vi "Actor Core.vi"(8 "error in":errorcluster, 11 "Aumentar_contador in":refnum<class "Aumentar_contador.lvclass">) -> (0 "error out":errorcluster, 3 "Actor out":refnum<class "Actor.lvclass">)   [LabVIEW 2019, in "Aumentar_contador.lvlib" / "Aumentar_contador.lvclass"]
doc: "(<B>Filename</B>: Actor Framework.lvlib:Actor.lvclass:Actor Core.vi)\n\nReceives messages to the actor, reacts to them, and initiates any error handling that may shut the actor down.\n\nDescendant classes may override this VI to append parallel tasks for the actor to complete while it handles messages. Overrides use the Call Parent Method node."
uses:
  Aumentar_contador.lvclass
  C:/Program Files/National Instruments/LabVIEW 2019/vi.lib/ActorFramework/Actor/Actor.lvclass
  <vilib>/ActorFramework/Actor/Actor.lvclass
  <vilib>/ActorFramework/Actor/Actor.lvclass/Actor.ctl
  Aumentar_contador.lvclass/Aumentar_contador.ctl
  Contador_Bin_Actor Messages/Update_Cuenta Msg/Update_Cuenta Msg.lvclass/Update_Cuenta Msg.ctl
  <vilib>/ActorFramework/Message Enqueuer/Message Enqueuer.lvclass/Message Enqueuer.ctl
  <vilib>/ActorFramework/Message Enqueuer/Enqueue.vi
  Contador_Bin_Actor Messages/Update_Cuenta Msg/Update_Cuenta Msg.lvclass
  C:/Program Files/National Instruments/LabVIEW 2019/vi.lib/ActorFramework/Message/Message.lvclass
  <vilib>/ActorFramework/Message Priority Queue/Priority Enqueue.vi
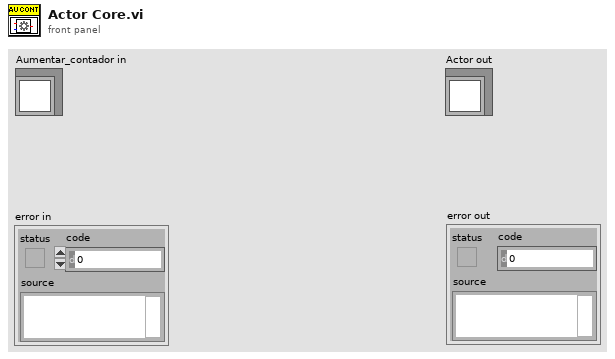
[diagram p1: front panel]
types:
  T1 = cluster{"Exit":refnum<user-event>, "Start/Stop":refnum<user-event>, "Lim. Inferior":refnum<user-event>, "Lim. Superior":refnum<user-event>}
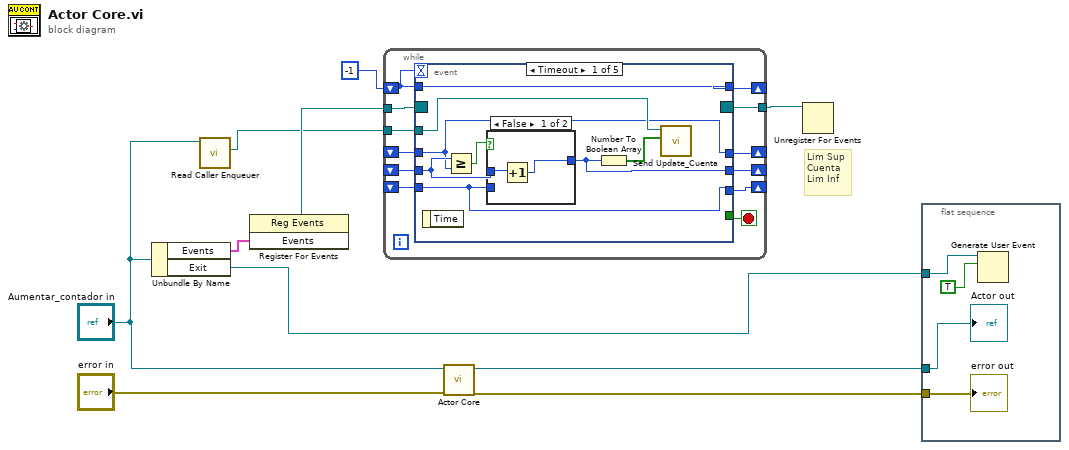
[diagram p0: block diagram]
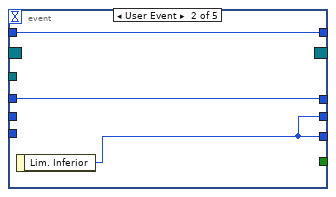
[diagram p3: hidden frame]
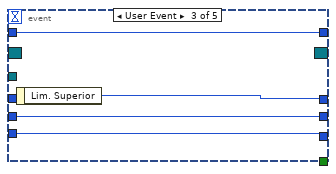
[diagram p4: hidden frame]
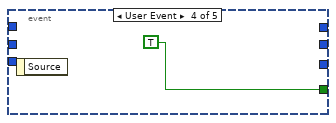
[diagram p5: hidden frame]
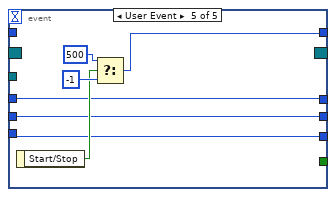
[diagram p6: hidden frame]
diagram:
  # "Lim Sup\nCuenta\nLim Inf"
  n1 = Unbundle By Name("Aumentar_contador in") -> ("Events"=w6:T1, "Exit"=w3:refnum<user-event>)
  n2 = call <vilib>:"Read Caller Enqueuer.vi"("Actor"="Aumentar_contador in") -> ("Caller Enqueuer"=w1:refnum<class "Message Enqueuer.lvclass">)  [unwired: 10 in]
  n3 = register-events(w6) -> (reference out=w5:refnum<event-registration>)  [unwired: 2 in, 1 out]
  n4 = while {
    shift-right: [w22] -> _
    shift-left: -1 -> [w21]
    tunnel: w5 -> [w20]
    tunnel: [w19] -> w4
    tunnel: w1 -> [w17]
    shift-right: [w16] -> _
    shift-left: _ -> [w15]
    shift-right: [w14] -> _
    shift-left: _ -> [w13]
    shift-right: [w12] -> _
    shift-left: _ -> [w11]
    stop <- w18 stop-if-true
    n5 = event shown="[0] Timeout" {
      selector: w20 -> [_ _ _ _ _]
      dyn-events: [_ _ _ _ _] -> w19
      timeout: w21 -> [_ _ _ _ _]
      tunnel: w21 -> [w30 w36 w38 _ _]
      tunnel: [w30 w36 w38 _ w46] -> w22
      tunnel: [_ _ _ TRUE _] -> w18
      tunnel: w17 -> [w29 _ _ _ _]
      tunnel: [w23 w34 w40 _ w42] -> w16
      tunnel: w15 -> [w23 _ w40 _ w42]
      tunnel: [w24 w35 w39 _ w44] -> w14
      tunnel: w13 -> [w24 w35 _ _ w44]
      tunnel: [w26 w34 w37 _ w43] -> w12
      tunnel: w11 -> [w25 _ w37 _ w43]
      event Timeout {
        n6 = event-data() -> ()  [unwired: 1 in, 1 out]
        n7 = Greater Or Equal?(x=w25, y=w24) -> (x >= y?=w27:bool)
        n8 = case shown="False" w27 {
          tunnel: [w31 w33] -> w26
          tunnel: w23 -> [_ w33]
          tunnel: w25 -> [w32 _]
          frame False {
            n9 = Increment(x=w32) -> (x+1=w31:u8)
          }
          frame True {
          }
        }
        n10 = Number To Boolean Array(number=w26) -> (Boolean array=w28:bool[])
        n11 = call "Send Update_Cuenta.vi"("Cuenta"=w28, "Message Enqueuer"=w29) -> ()  [unwired: 8 in, 2 out]
      }
      event User Event {
        n12 = event-data() -> ("Lim. Inferior"=w34:u8)  [unwired: 1 in]
      }
      event User Event {
        n13 = event-data() -> ("Lim. Superior"=w39:u8)  [unwired: 1 in]
      }
      event User Event {
        n14 = event-data() -> ()  [unwired: 1 in, 1 out]
      }
      event User Event {
        n15 = event-data() -> ("Start/Stop"=w45:bool)  [unwired: 1 in]
        n16 = Select(t=500, s=w45, f=-1) -> (s? t:f=w46:i32)
      }
    }
  }
  n17 = call-parent "Actor Core.vi"("error in"="error in", "Actor in"="Aumentar_contador in") -> ("error out"=w10:errorcluster, "Actor out"=w9:refnum<class "Actor.lvclass">)  [unwired: 8 in]
  n18 = Unregister For Events(event registration refnum=w4) -> ()  [unwired: 1 in, 1 out]
  n19 = flat-sequence {
    tunnel: w10 -> [w52]
    tunnel: w9 -> [w51]
    tunnel: w3 -> [w50]
    frame #0 {
      n20 = Generate User Event(user event=w50, event data cluster=TRUE ("event data")) -> ()  [unwired: 2 in, 2 out]
      "error out" <- w52
      "Actor out" <- w51
    }
  }
